vi "Filter Data Indeces.vi"(8 "error in (no error)":errorcluster, 10 "TimingGrp.lvclass":refnum<class "TimingGrp.lvclass">, 11 "Selected Group":refnum<class "ChanGrp.lvclass">) -> (0 "error out":errorcluster, 2 "MB Chan Indeces":i32[](array[numeric]), 3 "Selected Chan Indeces":i32[](array[numeric]))   [LabVIEW 2012, in "Configuration Grandmaster.lvlib" / "ChanGrp.lvclass"]
uses:
  ChanGrp.lvclass
  Class Timing Group/TimingGrp.lvclass
  ChanGrp.lvclass/ChanGrp.ctl
  Measurements/Class Channel/Read ChanName.vi
  Measurements/Class Channel/Read ToModBus.vi
  Measurements/Class Channel/Channel.lvclass
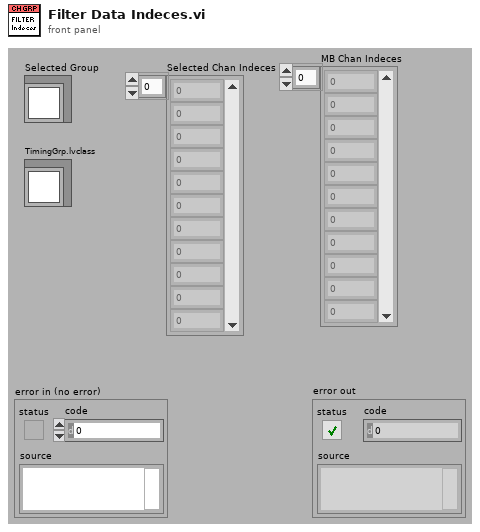
[diagram p1: front panel]
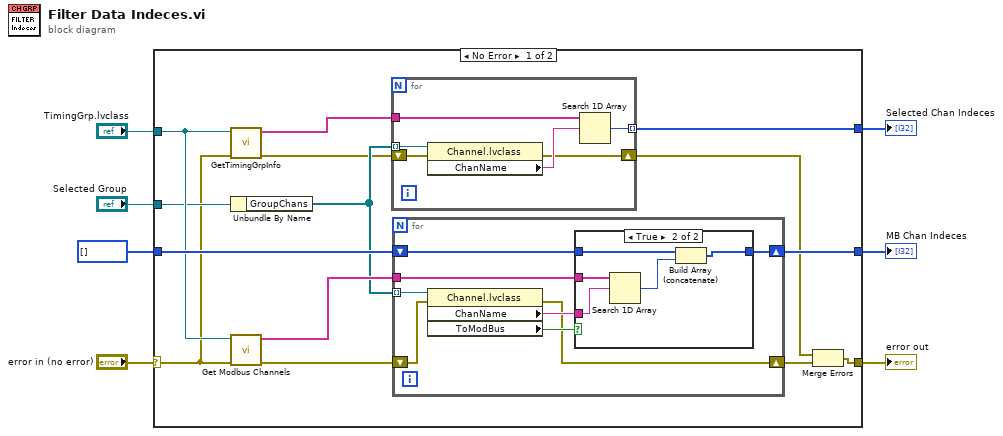
[diagram p0: block diagram]
diagram:
  n1 = case shown="No Error" "error in (no error)" {
    selector: "error in (no error)" -> [w8 w43]
    tunnel: [w21 w42] -> w7
    tunnel: i32[] [] -> [w19 w42]
    tunnel: [w18 w42] -> w5
    tunnel: "TimingGrp.lvclass" -> [w17 _]
    tunnel: "Selected Group" -> [w15 _]
    tunnel: [w9 w43] -> w2
    frame No Error {
      n2 = call "GetTimingGrpInfo.vi"("error in"=w8, "TimingGrp in"=w17) -> ("error out"=w13:errorcluster, "All TimingGrp Chans"=w16:string[])  [unwired: 4 in, 4 out]
      n3 = Unbundle By Name(w15) -> ("GroupChans"=w14:refnum<class "Channel.lvclass">[])
      n4 = call "Get Modbus Channels.vi"("error in (no error)"=w8, "TimingGrp.lvclass"=w17) -> ("error out"=w12:errorcluster, "All Rate MB Chans"=w20:string[])  [unwired: 7 in, 1 out]
      n5 = for {
        tunnel: w16 -> [w41]
        tunnel: [w40] -> w21 mode=indexing
        tunnel: w14 -> [w39] mode=indexing
        shift-right: [w36] -> w10
        shift-left: w13 -> [w37]
        n6 = property class="Channel.lvclass"(reference=w39, error in=w37) -> (error out=w36:errorcluster, "ChanName"=w38:string)  [unwired: 1 out]
        n7 = Search 1D Array(1D array=w41, element=w38) -> (index of element=w40:i32)  [unwired: 1 in]
      }
      n8 = for {
        tunnel: w20 -> [w29]
        tunnel: w14 -> [w26] mode=indexing
        shift-right: [w27] -> w18
        shift-left: w19 -> [w28]
        shift-right: [w23] -> w11
        shift-left: w12 -> [w22]
        n9 = property class="Channel.lvclass"(reference=w26, error in=w22) -> (error out=w23:errorcluster, "ChanName"=w24:string, "ToModBus"=w25:bool)  [unwired: 1 out]
        n10 = case shown="True" w25 {
          tunnel: w29 -> [_ w35]
          tunnel: w24 -> [_ w34]
          tunnel: w28 -> [w30 w33]
          tunnel: [w30 w31] -> w27
          frame False {
          }
          frame True {
            n11 = Search 1D Array(1D array=w35, element=w34) -> (index of element=w32:i32)  [unwired: 1 in]
            n12 = Build Array (concatenate)(w33, w32) -> (w31:i32[])
          }
        }
      }
      n13 = Merge Errors(w10, w11) -> (w9:errorcluster)
    }
    frame Error {
    }
  }
  "Selected Chan Indeces" <- w7
  "MB Chan Indeces" <- w5
  "error out" <- w2
